vi "set value_old.vi"(8 "error in (no error)":errorcluster, 9 "Set value":dbl, 10 "Control Name":string="Pre-Acc", 11 "VI Refnum":refnum<vi>) -> (0 "error out":errorcluster, 3 "Output string":string)   [LabVIEW 2016, in "sub-VIs.lvlib"]
doc: "Used to set value for control value of a given VI\n\nset scale_old.VI was used by Scale and Scale - Molecular. In PRIME Control 2017a, the R45 and Trans Quads have their set points communicated only on value-change events. The invoke node used in set scale_old.VI doesn't induce a value change events, so while the control value is changed, an event is not triggered and the value isn't communicated to power supply. The latest version (set scale.vi) uses property nodes and to set the control value via the Value Signalling property which does trigger an event."
uses:
  sub-VIs/sub-VIs.lvlib
panel:
  out "reference out":refnum<vi>
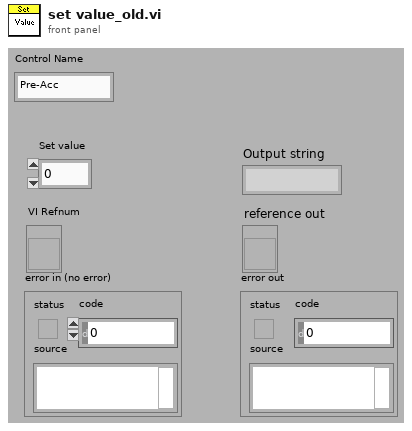
[diagram p1: front panel]
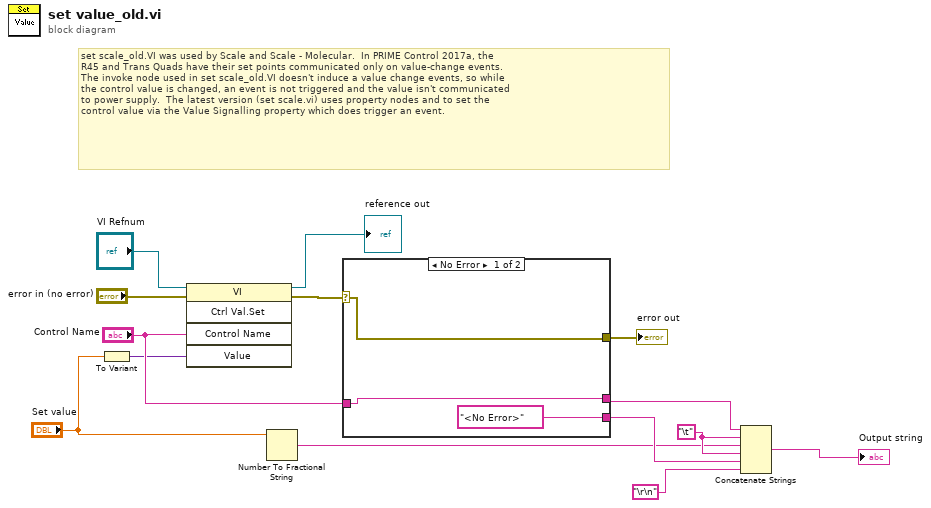
[diagram p0: block diagram]
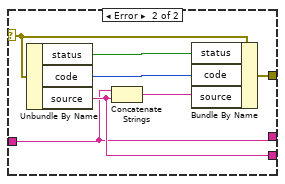
[diagram p2: hidden frame]
diagram:
  w10 = "\t"
  # "set scale_old.VI was used by Scale and Scale - Molecular.  In PRIME Control 2017a, the \nR45 and Trans Quads have their set points communicated only on value-change events.\nThe invoke node used in set scale_old.VI doesn't induce a value change events, so while \nthe control value is changed, an event is not triggered and the value isn't communicated \nto power supply.  The latest version (set scale.vi) uses property nodes and to set the \ncontrol value via the Value Signalling property which does trigger an event."
  n1 = To Variant(anything="Set value") -> (Variant=w2:variant)
  n2 = invoke class="VI" method="Ctrl Val.Set"(reference="VI Refnum", error in="error in (no error)", "Control Name"="Control Name", "Value"=w2) -> (reference out=→"reference out":refnum<vi>, error out=w12:errorcluster)  [unwired: 1 in, 3 out]
  n3 = Number To Fractional String(number="Set value") -> (F-format string=w5:string)  [unwired: 3 in]
  n4 = case shown="No Error" w12 {
    selector: w12 -> [w17 w24]
    tunnel: [w17 w21] -> w11
    tunnel: "Control Name" -> [w16 w18]
    tunnel: ["<No Error>" ("source") w19] -> w8
    tunnel: [w16 w18] -> w9
    frame No Error {
    }
    frame Error {
      n5 = Unbundle By Name(w24) -> ("status"=w23:bool, "code"=w22:i32, "source"=w19:string)
      n6 = Concatenate Strings(w18, w19) -> (w20:string)
      n7 = Bundle By Name(cluster=w24, "status"=w23, "code"=w22, "source"=w20) -> (w21:errorcluster)
    }
  }
  "error out" <- w11
  n8 = Concatenate Strings(w9, w10, w5, w10, w8, "\r\n") -> (→"Output string":string)
